vi "Validate_Create & Compile Functions.vi"(0 "scripts manager in":refnum<class "scripts manager.lvclass">, 5 "Functions in":T1[](array[typedef]), 11 "error in (no error)":errorcluster) -> (4 "scripts manager":refnum<class "scripts manager.lvclass">, 6 "Comiplation message":T2[](array[typedef]), 15 "error out":errorcluster)   [LabVIEW 2019, in "LSL.lvlib" / "scripts manager.lvclass"]
uses:
  scripts manager.lvclass
  common/function utils/Validate_message.ctl
  common/function utils/Validate_MessageStatus.ctl
  common/line and indent/Line Details.ctl
  scripts manager.lvclass/scripts manager.ctl
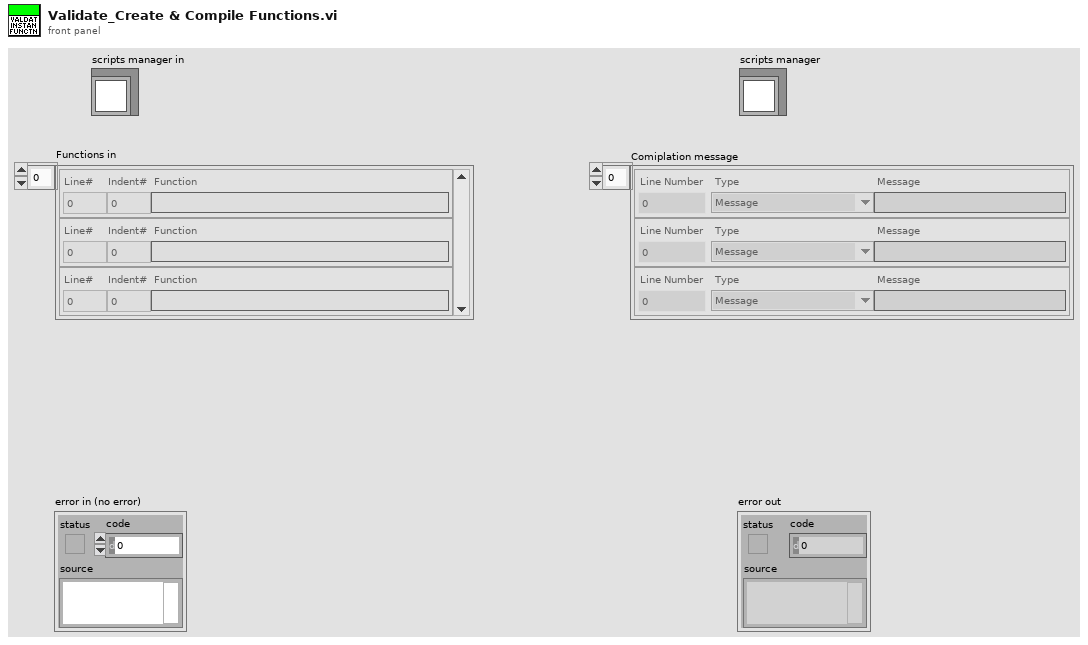
[diagram p1: front panel]
types:
  T1 = typedef "Line Details.ctl" = cluster{"Line#":i64, "Indent#":i64, "Function":string}
  T2 = typedef "Validate_message.ctl" = cluster{"Line Number":i64, "Type":T3, "Message":string}
  T3 = typedef "Validate_MessageStatus.ctl" = enum16{"Message", "Warning", "Error"}
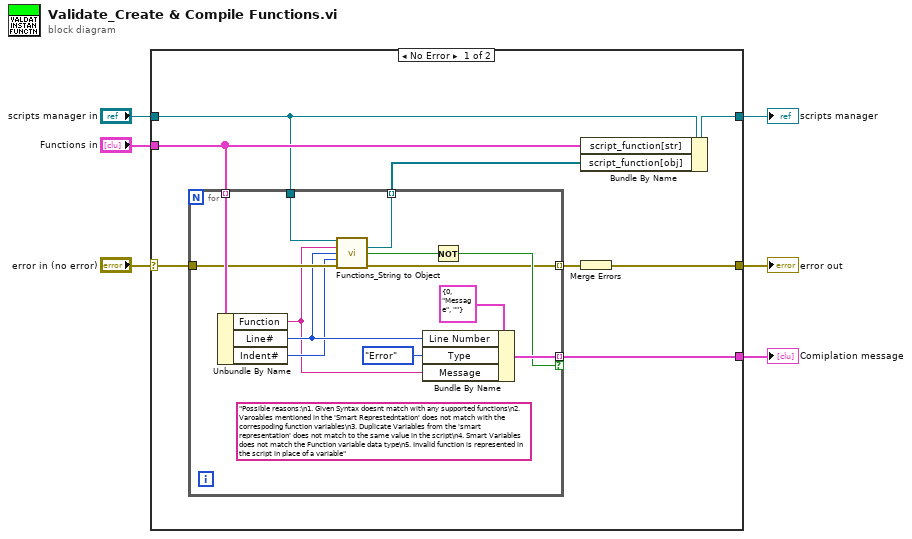
[diagram p0: block diagram]
diagram:
  n1 = case shown="No Error" "error in (no error)" {
    selector: "error in (no error)" -> [w14 w29]
    tunnel: [w12 w29] -> w5
    tunnel: [w11 _] -> w4
    tunnel: [w10 w28] -> w3
    tunnel: "scripts manager in" -> [w7 w28]
    tunnel: "Functions in" -> [w8 _]
    frame No Error {
      n2 = for {
        tunnel: w8 -> [w27] mode=indexing
        tunnel: w14 -> [w22]
        tunnel: [w20] -> w13 mode=indexing
        tunnel: [w19] -> w9 mode=indexing
        tunnel: [w25] -> w11 mode=indexing if=w24
        tunnel: w7 -> [w23]
        (unwired) "Possible reasons:\n1. Given Syntax doesnt match with any supported functions\n2. Varoables mentioned in the 'Smart Represtedntation' does not match with the correspoding function variables\n3. Duplicate Variables from the 'smart representation' does not match to the same value in the script\n4. Smart Variables does not match the Function variable data type\n5. Invalid function is represented in the script in place of a variable" ("Message")
        n3 = Unbundle By Name(w27) -> ("Function"=w15:string, "Line#"=w18:i64, "Indent#"=w17:i64)
        n4 = call-dynamic "Functions_String to Object.vi"("scripts manager in"=w23, "Functions"=w15, "Line#"=w18, "Indent#"=w17, "error in (no error)"=w22) -> ("function obj"=w19:refnum<class "functionbase.lvclass">, "function created"=w21:bool, "error out"=w20:errorcluster)  [unwired: 7 in, 1 out]
        n5 = Bundle By Name(cluster=T2 {"Line Number"=0, "Type"=enum."Message", "Message"=""} ("Message"), "Line Number"=w18, "Type"=Validate_MessageStatus."Error", "Message"=w15) -> (w25:T2)
        n6 = Not(x=w21) -> (.not. x?=w24:bool)
      }
      n7 = Bundle By Name(cluster=w7, "script_function[str]"=w8, "script_function[obj]"=w9) -> (w10:refnum<class "scripts manager.lvclass">)
      n8 = Merge Errors(w13) -> (w12:errorcluster)
    }
    frame Error {
    }
  }
  "error out" <- w5
  "Comiplation message" <- w4
  "scripts manager" <- w3
